vi "Msg.vi"(7 "jettl in":refnum<class "Actor.lvclass">, 11 "Event Create Msg in":refnum<class "Event Create Msg Strategy.lvclass">) -> (5 "jettl out":refnum<class "Actor.lvclass">)   [LabVIEW 2021, in "jettl.lvlib" / "Event Create.lvlib" / "Event Create Msg Strategy.lvclass"]
uses:
  Event Create Msg Strategy.lvclass
  jettl/Actor/Actor.lvclass
  Event Create/Event Create.lvclass
  Event Create Msg Strategy.lvclass/Event Create Msg Strategy.ctl
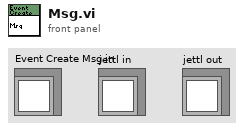
[diagram p1: front panel]
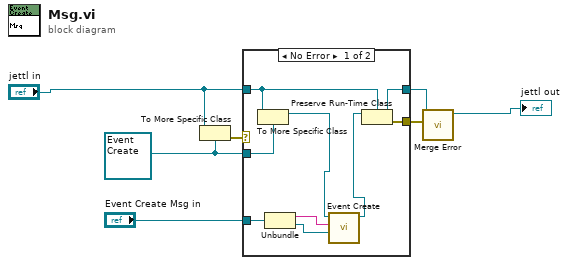
[diagram p0: block diagram]
diagram:
  w1 = refnum<class "Event Create.lvclass"> refnum ("Event Create.lvlib:Event Create.lvclass")
  n1 = To More Specific Class(target class=w1, reference="jettl in") -> (error out=w7:errorcluster)  [unwired: 1 in, 1 out]
  n2 = case shown="No Error" w7 {
    selector: w7 -> [_ w17]
    tunnel: [w14 w18] -> w5
    tunnel: "jettl in" -> [w15 w18]
    tunnel: w1 -> [w16 _]
    tunnel: [w13 w17] -> w6
    tunnel: "Event Create Msg in" -> [w10 _]
    frame No Error {
      n3 = To More Specific Class(target class=w16, reference=w15) -> (specific class reference=w11:refnum<class "Event Create.lvclass">)  [unwired: 1 in, 1 out]
      n4 = Unbundle(w10) -> (w9:string, w8:refnum<class "Event Actor.lvclass">)
      n5 = call-dynamic "Event Create.vi"("Event jettl"=w8, "Alias"=w9, "Event Create in"=w11) -> ("Event Create out"=w12:refnum<class "Event Create.lvclass">)  [unwired: 8 in]
      n6 = Preserve Run-Time Class(object in=w12, 2:w15) -> (object out=w14:refnum<class "Actor.lvclass">, error out=w13:errorcluster)  [unwired: 1 in]
    }
    frame Error {
    }
  }
  n7 = call-dynamic "Merge Error.vi"("Error"=w6, "Set Error in"=w5) -> ("Set Error out"=→"jettl out":refnum<class "Actor.lvclass">)  [unwired: 9 in]
